vi "Curtin1.vi"() -> ()   [LabVIEW 2022 SP3]
uses:
  ViolinSubs/Curtin1_Label.ctl
  ViolinSubs/GraphType.ctl
  <vilib>/Utility/miscctls.llb/LVPoint32TypeDef.ctl
  ViolinSubs/Mic/Mic_Global.vi
  ViolinSubs/Perspective/subs/Perspective_Globals.vi
  <vilib>/Platform/browser.llb/Open URL in Default Browser (string).vi
panel:
  in  "microphone":bool
  in  "Device":u16(ring) items=["BuerginBase Microphone", "MacBook Pro Microphone", "Microsoft Teams Audio"]
  out "comma?":bool
  out "startX":i32
  out "Ctrl":bool
  out "beta":string
  in  "Settings":u16(ring) items=["Settings...", "Preferences", "Templates", "Calibrations", "Live View", "Motor Cntrl"]
  in  "ScratchPads":u16(ring) items=["Scratch...", "Admittance Scratchpad", "Radiation ScratchPad", "ScratchPad", "TapTones ScratchPad"]
  in  "New Test":u16(ring) items=["New Test...", "Admittance H", "JC H 12 radiation", "JC H 7 radiation", "JC HV 24 radiation", "TEST"]
  in  "Help":bool
  in  "About":bool
  in  "Start":bool
  in  "email":bool
  in  "Interpret":bool
  in  "Force YRescale":bool
  out "Complex Out":cluster{dbl, "df":dbl, cdb[]}[](array[cluster])
  out "# selected":i32
  in  "Fun":bool
  out "Version":string
  in  "Preferences":bool
  in  "Set Colors":bool
  in  "Colors":u16(ring) items=["Name Current...", "Last Saved", "24 Colors", "rear"]
  in  "Share":bool
  in  "Undo":bool
  in  "Clear All":bool
  in  "select all":bool
  in  "deselect":bool
  in  "Clear":bool
  in  "Lists":bool
  in  "Browse":bool
  in  "Search":bool
  in  "Redo":bool
  in  "Files":T1[](array[typedef])
  in  "zoom":bool
  in  "Mouse Down?":bool
  in  "Views":T3={"View Type"=0, "Smoothing"=0, "Bands"=0, "Edit"=FALSE, "rescale Y"=FALSE, "rescale X"=FALSE, "X_Low"=0.0, "X_High"=0.0, "dB Range"=40.0, "Excel"=FALSE, "Y Scaling"=TRUE, "X Scaling"=TRUE, "Plot"=0} {"Plot" items=["FRF", "rad phase unwrapped", "deg phase unwrapped", "rad phase wrapped", "deg phase wrapped", "White Plots", "MJ Map", "Real and Imaginary"]; "Bands" items=["No Bands", "JC violin 200-7000 Flat (200-7000)", "JC violin (200-780-1740-2930-7000)", "JC violin (200-780-7000)"]; "Smoothing" items=["No smoothing"=0, "1/4 semitone"=25, "1/2 semitone"=50, "1 semitone"=100, "2 semitones"=200, "3 semitones"=300, "4 semitones"=400, "Octave"=1200, "Woodhouse"=19]; "View Type" items=["As measured"=0, "Normalize"=1, "Cplx Average"=3, "Real Average"=4, "Standard Deviation"=5]}
  out "Position":string
  in  "Color Table":T4(ring)=enum."Greyscale"
  out "MJPlot":dbl[][](graph)
  out "Coords":T5
  out "White Plots":picture
  out "FRF":cluster{"x0":dbl, "df":dbl, dbl[]}[](graph)
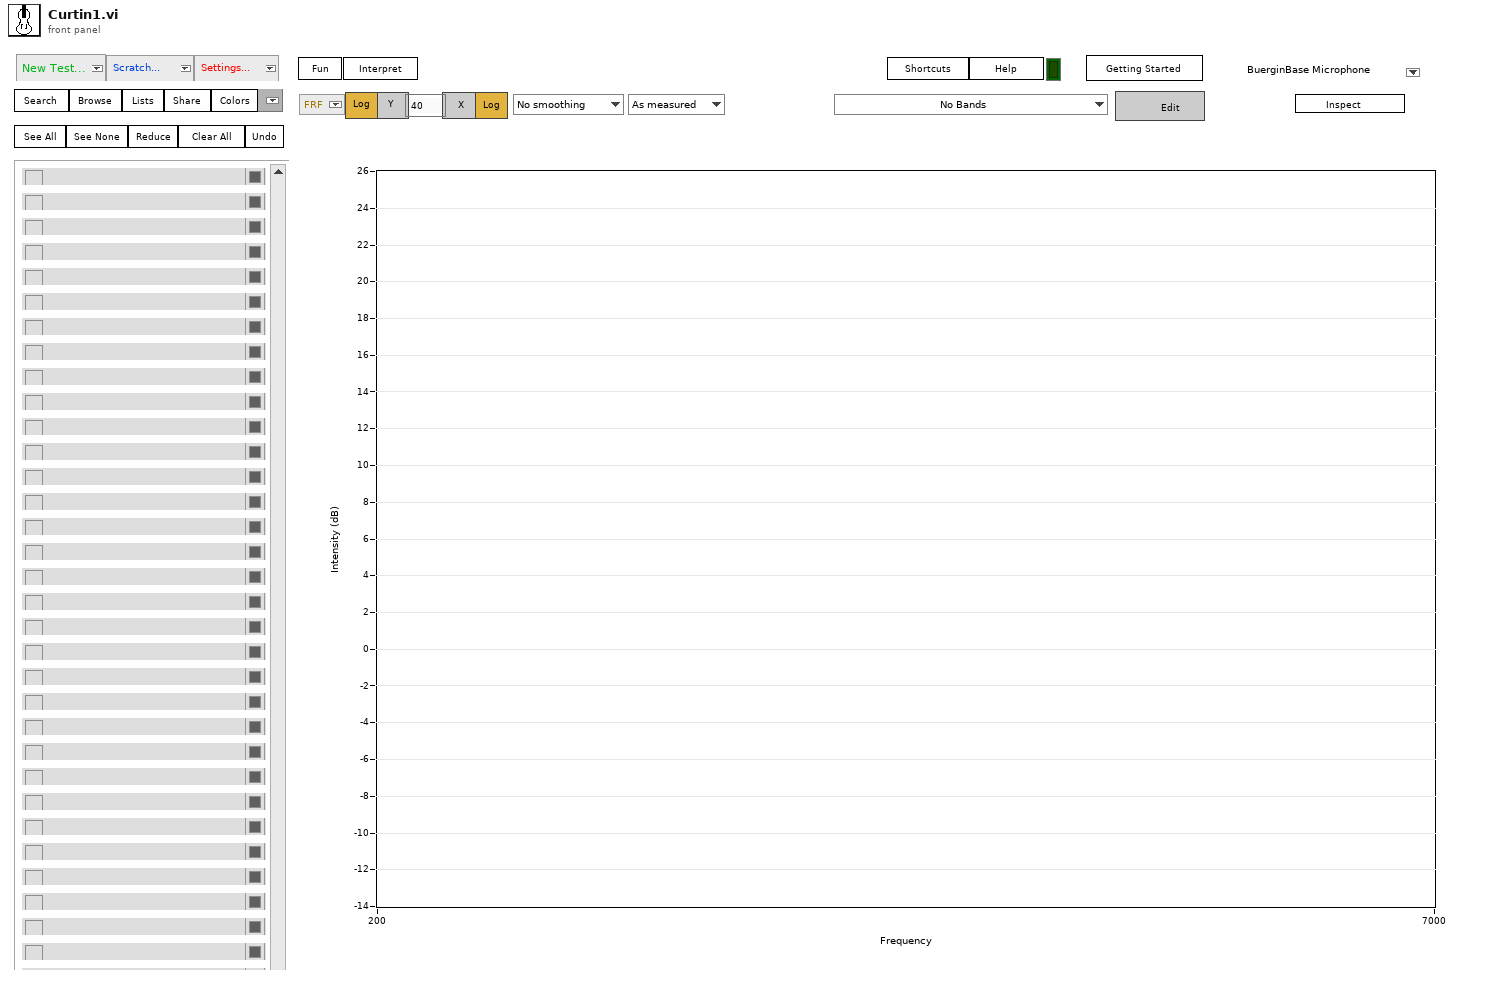
[diagram p1: front panel]
types:
  T1 = typedef "Curtin1_Label.ctl" = cluster{"Show?":bool, "Name":string, "Color":u32, "Path":path, "Show Notes":bool}
  T2 = typedef "GraphType.ctl" = u16
  T3 = cluster{"View Type":u16, "Smoothing":u16, "Bands":u16, "Edit":bool, "rescale Y":bool, "rescale X":bool, "X_Low":dbl, "X_High":dbl, "dB Range":dbl, "Excel":bool, "Y Scaling":bool, "X Scaling":bool, "Plot":T2}
  T4 = enum16{"Apricot", "Carnation", "Ether", "Greyscale", "Greyscale-banded", "Hot Metal", "Lava Waves", "Mac", "Morning Glory", "Rainbow", "Rainbow-banded", "Rainbow-inverted", "Rainbow-striped", "Saturn", "Seismic", "Space"}
  T5 = typedef "LVPoint32TypeDef.ctl" = cluster{"Horizontal":i32, "Vertical":i32}
  T6 = enum32{"SPL", "Voltage", "Accelerometer", "Vibrometer", "home", "Units"}
  T7 = enum16{"big-endian, network order", "native, host order", "little-endian"}
  T8 = enum16{"Grab Lines", "Grab Bands", "Grab Centroids"}
  T9 = cluster{"Alerts":bool, "Log X Axis":bool, "dB scale":bool, "Averaging":bool, "Fade":dbl, "Centroids?":bool}
  T10 = typedef "LVBoundsTypeDef.ctl" = cluster{"Width":u32, "Height":u32}
  T11 = typedef "LVPositionTypeDef.ctl" = cluster{"Left":i32, "Top":i32}
  T12 = typedef "PreferencesControl.ctl" = cluster{"Name of test":string, "Date":timestamp, "Location":string, "Template":string, "Soundcard":string, "resolution":u16, "Sampling rate":u16, "Ch1 Gain ":dbl, "Ch2 Gain":dbl, "Sample time (s)":dbl, "Pre-trigger (s)":dbl, "Hammer Threshold":dbl, "Positions":i16, "Taps/Position":i16, "Set Names":string, "Freq resolution":dbl, "Hammer cutoff":dbl, "Mic cutoff":dbl, "Double bounce ":dbl, "Hammer Cal":dbl, "dB Offset":dbl, "Accel Cal":dbl, "Vibrometer Cal":dbl, "Mic Cal":dbl, "Output":u16, "Voltage Cal":dbl, "Vibrometer Port":refnum<visa-resource-name>, "Range":u16, "High Pass":u16, "Bandwidth":u16, "X Range":cluster{"Minimum":dbl, "Maximum":dbl, "Increment":dbl, "Minor Increment":dbl, "Start":dbl}[], "Y Range":cluster{"Minimum":dbl, "Maximum":dbl, "Increment":dbl, "Minor Increment":dbl, "Start":dbl}[], "dB Spread":dbl, "Trigger":u16, "Ch_1":u8, "Ch_2":u8, "flip?":bool, "60Hz":bool, "Time offset":dbl, "Piezo Cal":dbl, "Default Notes":string}
  T13 = typedef "eventvkey.ctl" = enum16{"ASCII", "Enter", "Return", "Shift", "Ctrl", "Alt", "Cmd", "Opt", "Caps", "NumLock", "Clear", "Break", "Up", "Down", "Left", "Right", "Insert", "Delete", "Home", "End", "PageUp", "PageDown", "Escape", "Help", "Pause", "ScrollLock", "F1", "F2", "F3", "F4", "F5", "F6", "F7", "F8", "F9", "F10", "F11", "F12", "F13", "F14", "F15", "F16", "F17", "F18", "F19", "F20", "F21", "F22", "F23", "F24", "Play", "VolumeUp", "VolumeDown", "Mute", "Two Byte Char"}
  T14 = typedef "LVMouseTypeDef.ctl" = cluster{"Mouse Position":cluster{"X":i32, "Y":i32}, "Mouse Modifiers":cluster{"Button Down":bool, "Shift Mod":bool, "Menu Mod":bool, "Option Mod":bool}}
  T15 = enum32{"Invalid", "Standard", "Closed", "Hidden", "Minimized", "Maximized"}
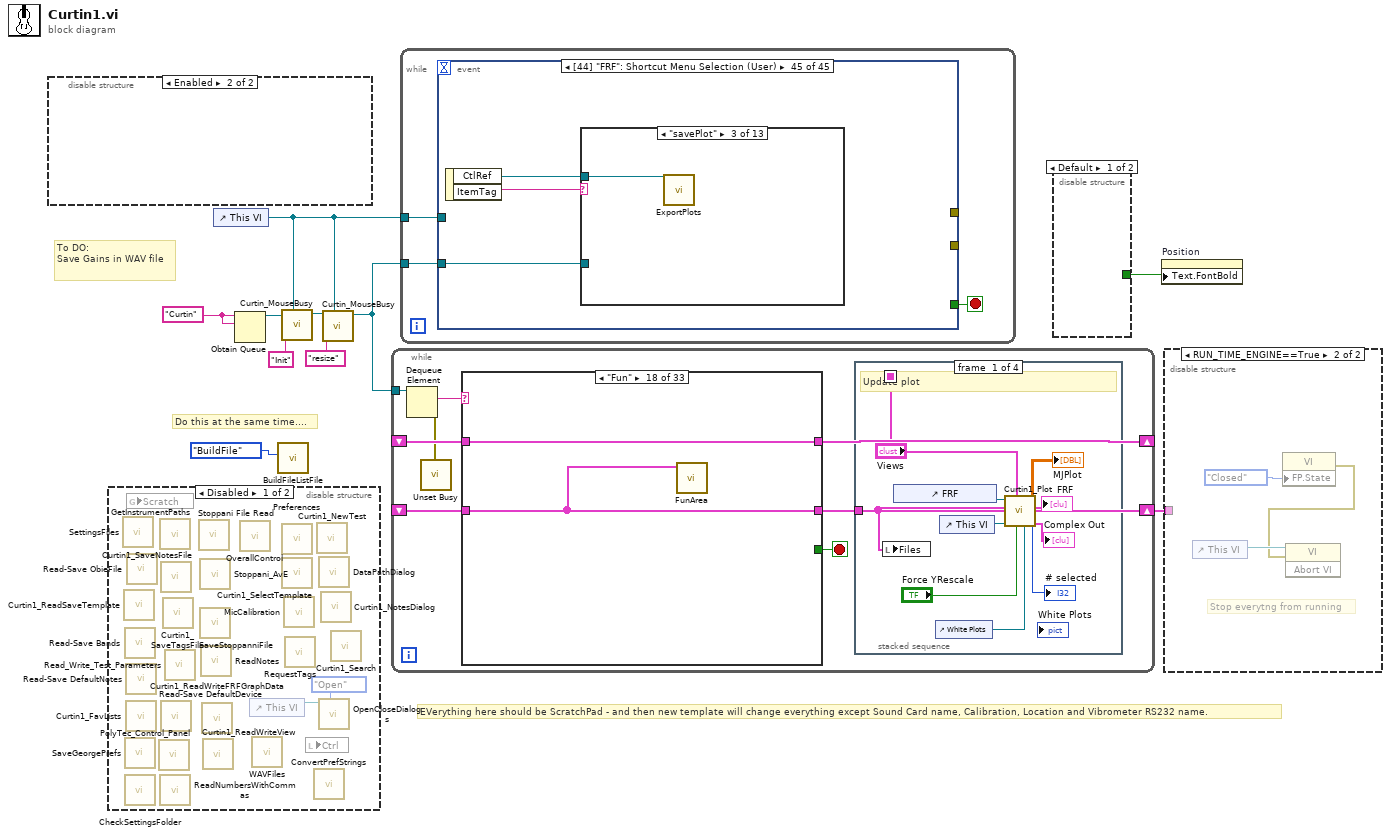
[diagram p0: block diagram]
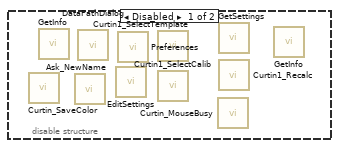
[diagram p2: hidden frame]
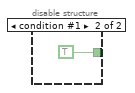
[diagram p4: hidden frame]
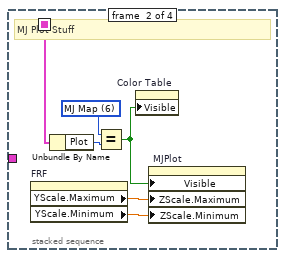
[diagram p6: hidden frame]
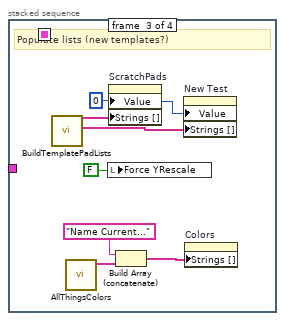
[diagram p7: hidden frame]
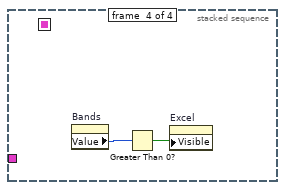
[diagram p8: hidden frame]
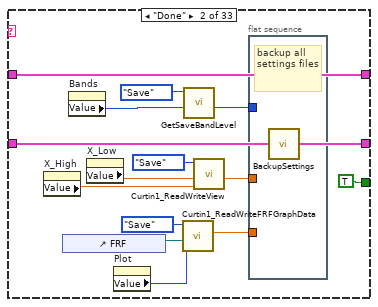
[diagram p10: hidden frame]
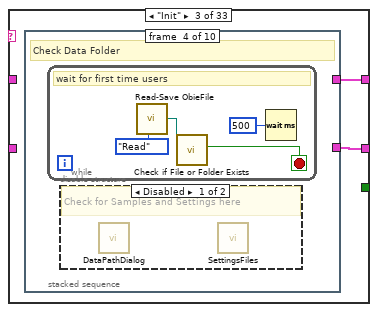
[diagram p11: hidden frame]
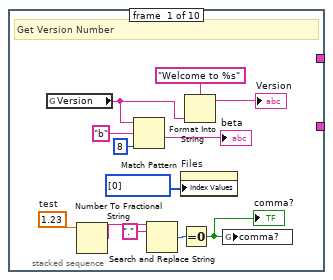
[diagram p12: hidden frame]
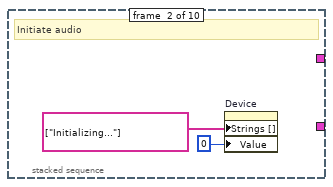
[diagram p13: hidden frame]
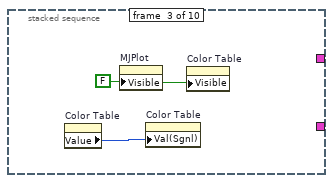
[diagram p14: hidden frame]
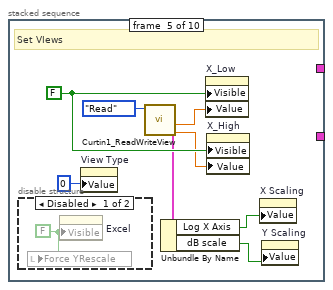
[diagram p16: hidden frame]
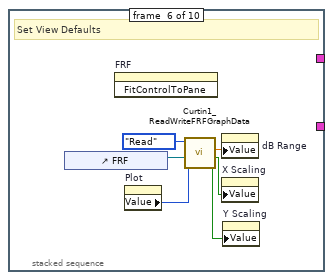
[diagram p18: hidden frame]
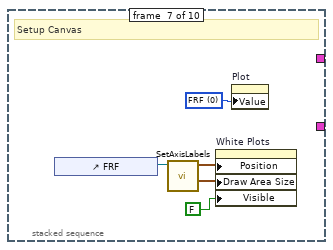
[diagram p19: hidden frame]
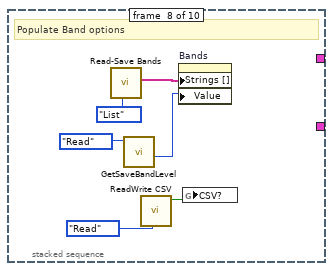
[diagram p20: hidden frame]
diagram:
  w8 = "Curtin" ("name (unnamed)")
  # "Do this at the same time...."
  # "To DO:\nSave Gains in WAV file"
  # "EVerything here should be ScratchPad - and then new template will change everything except Sound Card name, Calibration, Location and Vibrometer RS232 name."
  n1 = disable-structure shown="Enabled" {
    frame Disabled {
      n2 = call "Curtin_SaveColor.vi"() -> ()  [unwired: 10 in, 2 out]
      n3 = call "GetInfo.vi"() -> ()  [unwired: 11 in, 1 out]
      n4 = call "Ask_NewName.vi"() -> ()  [unwired: 10 in, 2 out]
      n5 = call "DataPathDialog.vi"() -> ()  [unwired: 10 in, 2 out]
      n6 = call "EditSettings.vi"() -> ()  [unwired: 10 in, 2 out]
      n7 = call "Preferences.vi"() -> ()  [unwired: 9 in, 3 out]
      n8 = call "Curtin1_SelectTemplate.vi"() -> ()  [unwired: 10 in, 2 out]
      n9 = call "Curtin1_SelectCalib.vi"() -> ()  [unwired: 11 in, 1 out]
      n10 = call "Curtin_MouseBusy.vi"() -> ()  [unwired: 11 in, 1 out]
      n11 = call "GetSettings.vi"() -> ()  [unwired: 10 in, 2 out]
      n12 = call "Curtin1_Recalc.vi"() -> ()  [unwired: 12 in]
      n13 = call "GetInfo.vi"() -> ()  [unwired: 11 in, 1 out]
    }
    frame Enabled {
    }
  }
  n14 = disable-structure shown="Disabled" {
    frame Disabled {
      n15 = call "SettingsFiles.vi"() -> ()  [unwired: 10 in, 2 out]
      n16 = call "Curtin1_ReadSaveTemplate.vi"() -> ()  [unwired: 8 in, 4 out]
      n17 = call "Read-Save Bands.vi"() -> ()  [unwired: 8 in, 4 out]
      n18 = call "SaveGeorgePrefs.vi"() -> ()  [unwired: 10 in, 2 out]
      n19 = call "CheckSettingsFolder.vi"() -> ()  [unwired: 12 in]
      n20 = call "Read-Save DefaultNotes.vi"() -> ()  [unwired: 10 in, 2 out]
      n21 = call "Curtin1_FavLists.vi"() -> ()  [unwired: 8 in, 4 out]
      n22 = global read "Mic_Global.vi" "Scratch"() -> ()  [unwired: 1 in]
      n23 = call "Read-Save ObieFile.vi"() -> ()  [unwired: 9 in, 3 out]
      n24 = call "PolyTec_Control_Panel.vi"() -> ()  [unwired: 9 in, 3 out]
      n25 = call "GetInstrumentPaths.vi"() -> ()  [unwired: 7 in, 5 out]
      n26 = call "ReadNumbersWithCommas.vi"() -> ()  [unwired: 8 in, 4 out]
      n27 = call "Curtin1_SaveNotesFile.vi"() -> ()  [unwired: 12 in]
      n28 = call "Read-Save DefaultDevice.vi"() -> ()  [unwired: 10 in, 2 out]
      n29 = call "Curtin1_SaveTagsFile.vi"() -> ()  [unwired: 12 in]
      n30 = call "Read_Write_Test_Parameters.vi"() -> ()  [unwired: 10 in, 2 out]
      n31 = call "Stoppani File Read.vi"() -> ()  [unwired: 3 in, 4 out]
      n32 = call "Stoppani_AvE.vi"() -> ()  [unwired: 8 in, 4 out]
      n33 = call "SaveStoppanniFile.vi"() -> ()  [unwired: 11 in, 1 out]
      n34 = call "ReadNotes.vi"() -> ()  [unwired: 10 in, 2 out]
      n35 = call "Curtin1_ReadWriteFRFGraphData.vi"() -> ()  [unwired: 9 in, 3 out]
      n36 = call "Curtin1_ReadWriteView.vi"() -> ()  [unwired: 9 in, 3 out]
      n37 = call "OverallControl.vi"() -> ()  [unwired: 10 in, 2 out]
      n38 = control-ref of="This VI"() -> (w11:refnum<vi>)
      n39 = call "WAVFiles.vi"() -> ()  [unwired: 8 in, 4 out]
      n40 = call "Preferences.vi"() -> ()  [unwired: 9 in, 3 out]
      n41 = call "Curtin1_SelectTemplate.vi"() -> ()  [unwired: 10 in, 2 out]
      n42 = call "MicCalibration.vi"() -> ()  [unwired: 11 in, 1 out]
      n43 = call "RequestTags.vi"() -> ()  [unwired: 11 in, 1 out]
      n44 = local read "Ctrl"() -> ()  [unwired: 1 in]
      n45 = call "ConvertPrefStrings.vi"() -> ()  [unwired: 10 in, 2 out]
      n46 = call "Curtin1_NewTest.vi"() -> ()  [unwired: 10 in, 2 out]
      n47 = call "DataPathDialog.vi"() -> ()  [unwired: 10 in, 2 out]
      n48 = call "OpenCloseDialogs.vi"("Task"=enum16{"Open", "Close"}."Open", "VI in"=w11) -> ()  [unwired: 8 in, 2 out]
      n49 = call "Curtin1_NotesDialog.vi"() -> ()  [unwired: 9 in, 3 out]
      n50 = call "Curtin1_Search.vi"() -> ()  [unwired: 10 in, 2 out]
    }
    frame Enabled {
    }
  }
  n51 = control-ref of="This VI"() -> (w2:refnum<vi>)
  n52 = Obtain Queue(name (unnamed)=w8, element data type=w8) -> (queue out=w7:refnum<queue>)  [unwired: 3 in, 2 out]
  n53 = call "BuildFileListFile.vi"("Task"=enum16{"BuildFile", "ReadFile"}."BuildFile") -> ()  [unwired: 9 in, 2 out]
  n54 = call "Curtin_MouseBusy.vi"("VI in"=w2, "element"="Init", "queue in"=w7) -> ("queue out"=w4:refnum<queue>)  [unwired: 8 in]
  n55 = call "Curtin_MouseBusy.vi"("VI in"=w2, "element"="resize", "queue in"=w4) -> ("queue out"=w5:refnum<queue>)  [unwired: 8 in]
  n56 = while {
    tunnel: w5 -> [w19]
    shift-right: [w16] -> w9
    shift-left: _ -> [w17]
    shift-right: [w14] -> _
    shift-left: _ -> [w15]
    stop <- w18 stop-if-true
    n57 = Dequeue Element(queue=w19) -> (element=w20:string, error out=w13:errorcluster)  [unwired: 2 in, 2 out]
    n58 = call <vilib>:"Unset Busy.vi"("error in (no error)"=w13) -> ()  [unwired: 10 in, 1 out]
    n59 = case shown="\"Fun\"" w20 {
      selector: w20 -> [_ _ _ _ _ _ _ _ _ _ _ _ _ _ _ _ _ _ _ _ _ _ _ _ _ _ _ _ _ _ w300 _ _]
      tunnel: [_ TRUE ("Discard?") _ _ _ _ _ _ _ _ _ _ _ _ _ _ _ _ _ _ _ _ _ _ _ _ _ _ _ _ _ _ _] -> w18
      tunnel: w17 -> [w47 w60 _ _ w128 w137 w153 w158 w160 w162 w164 w177 w184 w189 w200 w209 w221 w225 w227 w229 w233 w238 w241 w244 w257 w269 w275 w280 w285 w290 w301 w308 w331]
      tunnel: [w47 w60 w62 w116 w128 w139 w153 w158 w160 w162 w168 w176 w185 w191 w195 w209 w220 w225 w227 w229 w231 w237 w240 w244 w256 w268 w274 w282 T1[] [] ("Files") w292 w301 w308 w331] -> w16
      tunnel: [w46 w59 w63 w117 w131 w141 w154 w159 w161 w163 w166 w178 w186 w192 w201 w210 w223 w226 w228 w230 w234 w239 w242 w245 w258 w267 w273 w279 w286 w293 w302 w312 w332] -> w14
      tunnel: w15 -> [w46 w59 _ w118 w131 w141 w154 w159 w161 w163 w167 w179 w187 w193 w202 w210 w224 w226 w228 w230 w235 w239 w242 w245 w259 w267 w273 w281 w288 w291 w302 w312 w332]
      frame Default {
      }
      frame "Done" {
        n60 = property on="X_High" class="DigNum (strict)"() -> ("Value"=w54:dbl)  [unwired: 2 in, 2 out]
        n61 = control-ref of="FRF"() -> (w57:refnum<vi>)
        n62 = property on="Bands" class="Ring (strict)"() -> ("Value"=w52:u16)  [unwired: 2 in, 2 out]
        n63 = property on="X_Low" class="DigNum (strict)"() -> ("Value"=w55:dbl)  [unwired: 2 in, 2 out]
        n64 = property on="Plot" class="Ring (strict)"() -> ("Value"=w48:T2)  [unwired: 2 in, 2 out]
        n65 = call "Curtin1_ReadWriteFRFGraphData.vi"("Type"=w48, "FRF"=w57, "Task"=enum16{"Read", "Save"}."Save") -> ("dB"=w49:dbl)  [unwired: 6 in, 2 out]
        n66 = call "GetSaveBandLevel.vi"("Value in"=w52, "Task"=enum16{"Read", "Save"}."Save") -> ("Value out"=w51:u16)  [unwired: 9 in]
        n67 = call "Curtin1_ReadWriteView.vi"("X_High"=w54, "X_Low"=w55, "Task"=enum16{"Read", "Save"}."Save") -> ("X_Low out"=w50:dbl)  [unwired: 6 in, 2 out]
        n68 = flat-sequence {
          tunnel: w51 -> [_]
          tunnel: w50 -> [_]
          tunnel: w49 -> [_]
          frame #0 {
            # "backup all settings files"
            n69 = call "BackupSettings.vi"() -> ()  [unwired: 12 in]
          }
        }
      }
      frame "Init" {
        n70 = stacked-sequence {
          tunnel: [_ _ _ _ _ _ _ _ _ cluster{"files":T1[]}[] [] ("Array in")] -> w63
          tunnel: [_ _ _ _ _ _ _ _ _ T1[] [] ("Files")] -> w62
          frame #0 {
            w65 = 1.23  # test
            # "Get Version Number"
            n71 = global read "Mic_Global.vi" "Version"() -> (w69:string)
            n72 = Number To Fractional String(number=w65) -> (F-format string=w64:string)  [unwired: 3 in]
            n73 = Match Pattern(string=w69, regular expression="b", offset (0)=8) -> (after substring=→"beta":string)  [unwired: 3 out]
            n74 = Search and Replace String(input string=w64, search string=".") -> (number of replacements=w68:i32)  [unwired: 6 in, 3 out]
            n75 = property on="Files" class="Arr"("Index Values"=u32[] [0]) -> ()  [unwired: 2 in, 2 out]
            n76 = Equal To 0?(x=w68) -> (x = 0?=w66:bool)
            "comma?" <- w66
            n77 = Format Into String(format string="Welcome to %s", w69) -> (resulting string=→"Version":string)  [unwired: 2 in, 1 out]
            n78 = global write "Mic_Global.vi" "comma?"(w66) -> ()
          }
          frame #1 {
            # "Initiate audio"
            n79 = property on="Device" class="Ring (strict)"("Strings []"=string[] ["Initializing..."] ("Strings [4]"), "Value"=0) -> ()  [unwired: 2 in, 2 out]
          }
          frame #2 {
            w79 = FALSE ("Visible")
            n80 = property on="Color Table" class="Enum (strict)"() -> ("Value"=w78:T4)  [unwired: 2 in, 2 out]
            n81 = property on="MJPlot" class="IntGraph (strict)"("Visible"=w79) -> ()  [unwired: 2 in, 2 out]
            n82 = property on="Color Table" class="Enum (strict)"("Val(Sgnl)"=w78) -> ()  [unwired: 2 in, 2 out]
            n83 = property on="Color Table" class="Enum (strict)"("Visible"=w79) -> ()  [unwired: 2 in, 2 out]
          }
          frame #3 {
            # "Check Data Folder"
            n84 = while {
              stop <- w81 stop-if-true
              # "wait for first time users"
              n85 = call "Read-Save ObieFile.vi"("Task"=enum16{"Save", "Read"}."Read") -> ("DataPath Out"=w83:path)  [unwired: 8 in, 2 out]
              n86 = call <vilib>:"Check if File or Folder Exists.vi"("path"=w83) -> ("file or folder exists?"=w81:bool)  [unwired: 8 in, 2 out]
              n87 = Wait (ms)(milliseconds to wait=u32 500) -> ()  [unwired: 1 out]
            }
            n88 = disable-structure shown="Disabled" {
              frame Disabled {
                # "Check for Samples and Settings here"
                n89 = call "DataPathDialog.vi"() -> ()  [unwired: 10 in, 2 out]
                n90 = call "SettingsFiles.vi"() -> ()  [unwired: 10 in, 2 out]
              }
              frame Enabled {
              }
            }
          }
          frame #4 {
            w91 = FALSE ("Visible")
            # "Set VIews"
            n91 = disable-structure shown="Disabled" {
              frame Disabled {
                w92 = FALSE ("Visible")
                n92 = local write "Force YRescale"(w92) -> ()
                n93 = property on="Excel" class="Bool"("Visible"=w92) -> ()  [unwired: 2 in, 2 out]
              }
              frame Enabled {
              }
            }
            n94 = property on="View Type" class="Ring (strict)"("Value"=u16 0) -> ()  [unwired: 2 in, 2 out]
            n95 = call "Curtin1_ReadWriteView.vi"("Task"=enum16{"Read", "Save"}."Read") -> ("X_High out"=w88:dbl, "X_Low out"=w89:dbl, "View"=w84:T9)  [unwired: 8 in]
            n96 = Unbundle By Name(w84) -> ("Log X Axis"=w85:bool, "dB scale"=w86:bool)
            n97 = property on="X_Low" class="DigNum (strict)"("Visible"=w91, "Value"=w89) -> ()  [unwired: 2 in, 2 out]
            n98 = property on="X_High" class="DigNum (strict)"("Visible"=w91, "Value"=w88) -> ()  [unwired: 2 in, 2 out]
            n99 = property on="X Scaling" class="Bool (strict)"("Value"=w85) -> ()  [unwired: 2 in, 2 out]
            n100 = property on="Y Scaling" class="Bool (strict)"("Value"=w86) -> ()  [unwired: 2 in, 2 out]
          }
          frame #5 {
            # "Set View Defaults"
            n101 = control-ref of="FRF"() -> (w98:refnum<vi>)
            n102 = invoke on="FRF" class="WFGraph (strict)" method="FitControlToPane"() -> ()  [unwired: 3 in, 3 out]
            n103 = property on="Plot" class="Ring (strict)"() -> ("Value"=w95:T2)  [unwired: 2 in, 2 out]
            n104 = call "Curtin1_ReadWriteFRFGraphData.vi"("Type"=w95, "FRF"=w98, "Task"=enum16{"Read", "Save"}."Read") -> ("y log?"=w94:bool, "x log?"=w93:bool, "dB"=w96:dbl)  [unwired: 6 in]
            n105 = property on="dB Range" class="DigNum (strict)"("Value"=w96) -> ()  [unwired: 2 in, 2 out]
            n106 = property on="X Scaling" class="Bool (strict)"("Value"=w93) -> ()  [unwired: 2 in, 2 out]
            n107 = property on="Y Scaling" class="Bool (strict)"("Value"=w94) -> ()  [unwired: 2 in, 2 out]
          }
          frame #6 {
            w99 = T2 0 items=["FRF", "rad phase unwrapped", "deg phase unwrapped", "rad phase wrapped", "deg phase wrapped", "White Plots"] ("Value")
            # "Setup Canvas"
            n108 = control-ref of="FRF"() -> (w103:refnum<vi>)
            n109 = call "SetAxisLabels.vi"("WaveformGraph in"=w103) -> ("Bounds"=w101:T10, "Position"=w102:T11)  [unwired: 8 in, 1 out]
            n110 = property on="White Plots" class="Pict"("Position"=w102, "Draw Area Size"=w101, "Visible"=FALSE) -> ()  [unwired: 2 in, 2 out]
            n111 = property on="Plot" class="Ring (strict)"("Value"=w99) -> ()  [unwired: 2 in, 2 out]
          }
          frame #7 {
            # "Populate Band options"
            n112 = call "Read-Save Bands.vi"("Task"=enum16{"Save", "Read", "List"}."List") -> ("Long names"=w109:string[])  [unwired: 7 in, 3 out]
            n113 = call "GetSaveBandLevel.vi"("Task"=enum16{"Read", "Save"}."Read") -> ("Value out"=w106:u16)  [unwired: 10 in]
            n114 = call "ReadWrite CSV.vi"("Task"=enum16{"Save", "Read"}."Read") -> ("csv Out"=w104:bool)  [unwired: 10 in]
            n115 = property on="Bands" class="Ring (strict)"("Strings []"=w109, "Value"=w106) -> ()  [unwired: 2 in, 2 out]
            n116 = global write "Mic_Global.vi" "CSV?"(w104) -> ()
          }
          frame #8 {
            # "Always start everyone with ScratchPad \n\nRead the latest calibration but do not \ndo anything with it (no error code/saving)"
            # "Upload  ScratchPad template"
            n117 = call "UpdateScratchPad.vi"() -> ("Settings Out"=w111:T12)  [unwired: 10 in, 1 out]
            n118 = global write "Mic_Global.vi" "Settings"(w111) -> ()
            n119 = control-ref of="Device"() -> (w112:refnum<vi>)
            n120 = call "Curtin1_soundcards.vi"("hush?"=TRUE, "Settings In"=w111, "device:"=w112) -> ()  [unwired: 7 in, 2 out]
          }
          frame #9 {
            # "Initialize Undo and List"
          }
        }
      }
      frame "Update" {
        # "NOTE: info box is in this frame"
        n121 = call "Curtin1_NotesDialog.vi"("Files"="Files") -> ("Color"=w120:u32[], "removed?"=w119:bool, "Array"=w116:T1[])  [unwired: 8 in]
        n122 = call "Curtin1_Color.vi"("Color"=w120) -> ()  [unwired: 9 in, 2 out]
        n123 = case shown="True" w119 {
          tunnel: w118 -> [w122 w125]
          tunnel: [w122 w124] -> w117
          tunnel: w116 -> [_ w123]
          frame False {
          }
          frame True {
            # "removed a plot"
            n124 = call "Curtin_Undo.vi"("New Files"=w123, "Array in"=w125) -> ("Array out"=w124:cluster{"files":T1[]}[])  [unwired: 9 in]
          }
        }
        n125 = property on="Colors" class="Ring (strict)"("Value"=-1) -> ()  [unwired: 2 in, 2 out]
      }
      frame "Zoom" {
        n126 = for {
          tunnel: w128 -> [w134] mode=indexing
          tunnel: [w133] -> w127 mode=indexing if=w132
          n127 = Unbundle By Name(w134) -> ("Name"=w133:string, "Show?"=w132:bool)
        }
        n128 = property on="Plot" class="Ring (strict)"() -> ("Value"=w126:T2)  [unwired: 2 in, 2 out]
        n129 = property on="dB Range" class="DigNum (strict)"() -> ("Value"=w129:dbl)  [unwired: 2 in, 2 out]
        n130 = control-ref of="FRF"() -> (w130:refnum<vi>)
        n131 = call "GraphZoom.vi"("Plot"=w126, "Names"=w127, "dB Range"=w129, "Graph"=w130) -> ()  [unwired: 8 in]
      }
      frame "Preferences" {
        n132 = control-ref of="Files"() -> (w140:refnum<vi>)
        n133 = call "Preferences.vi"("FileList"=w140, "Files"=w137) -> ("Settings out"=w135:T12, "Success?"=w138:bool, "Fixed Files"=w136:T1[])  [unwired: 7 in]
        n134 = case shown="True" w138 {
          tunnel: w136 -> [_ w150]
          tunnel: [w142 w150] -> w139
          tunnel: w137 -> [w142 _]
          tunnel: w135 -> [_ w146]
          frame False {
          }
          frame True {
            n135 = global read "Mic_Global.vi" "View"() -> (w149:T9)
            n136 = call "UpdateScratchPad.vi"("Settings"=w146) -> ("Settings Out"=w143:T12)  [unwired: 9 in, 1 out]
            n137 = Unbundle By Name(w149) -> ("Log X Axis"=w148:bool, "dB scale"=w147:bool)
            n138 = control-ref of="Device"() -> (w145:refnum<vi>)
            n139 = call "Curtin1_soundcards.vi"("hush?"=TRUE, "Settings In"=w143, "device:"=w145) -> ()  [unwired: 7 in, 2 out]
            n140 = property on="X Scaling" class="Bool (strict)"("Value"=w148) -> ()  [unwired: 2 in, 2 out]
            n141 = property on="Y Scaling" class="Bool (strict)"("Value"=w147) -> ()  [unwired: 2 in, 2 out]
          }
        }
      }
      frame "Templates" {
        n142 = global read "Mic_Global.vi" "Scratch"() -> (w152:string)
        n143 = call "EditSettings.vi"("Template in"=w152) -> ("Settings out"=w151:T12)  [unwired: 9 in, 1 out]
        n144 = call "UpdateScratchPad.vi"("Settings"=w151) -> ()  [unwired: 9 in, 2 out]
      }
      frame "Calibrations" {
        # "Saves a new calib file\nand it is pushed in test"
        n145 = call "UpdateScratchPad.vi"() -> ("Settings Out"=w156:T12)  [unwired: 10 in, 1 out]
        n146 = call "MicCalibration.vi"("Type"=T6."home" ("Tyoe"), "Settings"=w156) -> ("Settings Out"=w155:T12)  [unwired: 9 in]
        n147 = global write "Mic_Global.vi" "Settings"(w155) -> ()
        n148 = call "UpdateScratchPad.vi"("Settings"=w155) -> ()  [unwired: 9 in, 2 out]
      }
      frame "LiveView" {
        n149 = call "LiveSignal.vi"() -> ()  [unwired: 12 in]
      }
      frame "MotorControl" {
        n150 = call "MotorControl.vi"() -> ()  [unwired: 12 in]
      }
      frame "Browse" {
        n151 = Array Size(array=w164) -> (size(s)=w165:i32)
        n152 = case shown="0" w165 {
          frame Default {
          }
          frame 0 {
            n153 = local write "Force YRescale"(TRUE ("Force YRescale")) -> ()
          }
        }
        n154 = call "Curtin_Undo.vi"("New Files"=w164, "Array in"=w167) -> ("Array out"=w166:cluster{"files":T1[]}[])  [unwired: 9 in]
        n155 = call "Curtin1_LoadFile.vi"("Files in"=w164) -> ("Files out"=w168:T1[])  [unwired: 10 in]
      }
      frame "Preload" {
        n156 = call "Curtin1_GlobalFolder.vi"() -> ("Samples"=w170:path)  [unwired: 1 in, 1 out]
        n157 = List Folder(path=w170, pattern="*.AvC") -> (path out=w173:path, filenames=w172:string[])  [unwired: 2 in, 2 out]
        n158 = call "Curtin_Undo.vi"("New Files"=w177, "Array in"=w179) -> ("Array out"=w178:cluster{"files":T1[]}[])  [unwired: 9 in]
        n159 = local write "Force YRescale"(TRUE ("Force YRescale")) -> ()
        n160 = for {
          tunnel: w173 -> [w182]
          tunnel: w172 -> [w181] mode=indexing
          tunnel: [w180] -> w171 mode=indexing
          n161 = Build Path(base path=w182, name or relative path=w181) -> (appended path=w180:path)
        }
        n162 = call "Curtin1_AddTest.vi"("Selected Paths"=w171) -> ("New Files"=w176:T1[])  [unwired: 10 in]
      }
      frame "Search" {
        n163 = Array Size(array=w184) -> (size(s)=w183:i32)
        n164 = case shown="0" w183 {
          frame Default {
          }
          frame 0 {
            n165 = local write "Force YRescale"(TRUE ("Force YRescale")) -> ()
          }
        }
        n166 = call "Curtin_Undo.vi"("New Files"=w184, "Array in"=w187) -> ("Array out"=w186:cluster{"files":T1[]}[])  [unwired: 9 in]
        n167 = call "Curtin1_Search.vi"("Old Files"=w184) -> ("New Files"=w185:T1[])  [unwired: 9 in, 1 out]
      }
      frame "Lists" {
        n168 = Array Size(array=w189) -> (size(s)=w190:i32)
        n169 = case shown="0" w190 {
          frame Default {
          }
          frame 0 {
            n170 = local write "Force YRescale"(TRUE ("Force YRescale")) -> ()
          }
        }
        n171 = call "Curtin_Undo.vi"("New Files"=w189, "Array in"=w193) -> ("Array out"=w192:cluster{"files":T1[]}[])  [unwired: 9 in]
        n172 = call "Curtin1_Lists.vi"("Old Files"=w189) -> ("New Files"=w191:T1[])  [unwired: 10 in]
      }
      frame "newColors" {
        n173 = property on="Colors" class="Ring (strict)"() -> ("Strings []"=w198:string[], "Value"=w199:u16)  [unwired: 2 in, 2 out]
        n174 = Index Array(array=w198, index=w199) -> (element=w197:string)
        n175 = call "AllThingsColors.vi"("Choice"=w197) -> ("Possible Colors"=w196:string[])  [unwired: 10 in]
        n176 = for {
          tunnel: w200 -> [w206] mode=indexing
          tunnel: [w205] -> w195 mode=indexing
          tunnel: w196 -> [_]
          i -> [w204]
          n177 = call "Curtin1_Color.vi"("Offset"=w204) -> ("New color"=w203:u32)  [unwired: 9 in, 1 out]
          n178 = Bundle By Name(cluster=w206, "Color"=w203) -> (w205:T1)
        }
        n179 = call "Curtin_Undo.vi"("New Files"=w200, "Array in"=w202) -> ("Array out"=w201:cluster{"files":T1[]}[])  [unwired: 9 in]
        n180 = local write "Files"(w195) -> ()
      }
      frame "saveColors" {
        n181 = call "Curtin_SaveColor.vi"() -> ("New Color"=w208:string, "Good?"=w207:bool)  [unwired: 10 in]
        n182 = case shown="True" w207 {
          tunnel: w209 -> [_ w214]
          tunnel: w208 -> [_ w212]
          tunnel: [_ w213] -> _
          frame False {
          }
          frame True {
            n183 = for {
              tunnel: w214 -> [w219] mode=indexing
              tunnel: [w218] -> w217 mode=indexing
              n184 = Unbundle By Name(w219) -> ("Color"=w218:u32)
            }
            n185 = call "SettingsFiles.vi"("settings file name"=w212) -> ("file path"=w211:path)  [unwired: 9 in, 1 out]
            n186 = Write to Binary File(file (use dialog)=w211, data=w217, 5:FALSE ("prepend array or string size? (T)"), 9:T7."big-endian, network order" ("byte order (0:big-endian, network order)")) -> (error out=w213:errorcluster)  [unwired: 2 in, 2 out]
          }
        }
      }
      frame "setColors" {
        n187 = control-ref of="Files"() -> (w222:refnum<vi>)
        n188 = call "DefineColorPalette.vi"("Files in"=w221, "FileList"=w222) -> ("Files out"=w220:T1[])  [unwired: 9 in]
        n189 = call "Curtin_Undo.vi"("New Files"=w221, "Array in"=w224) -> ("Array out"=w223:cluster{"files":T1[]}[])  [unwired: 9 in]
      }
      frame "Fun" {
        n190 = call "FunArea.vi"("Old Files"=w225) -> ()  [unwired: 11 in]
      }
      frame "PlayIt" {
        n191 = call "PlayFile.vi"("Old Files"=w227) -> ()  [unwired: 11 in]
      }
      frame "Share" {
        n192 = call "Curtin1_Share.vi"("Files"=w229) -> ()  [unwired: 11 in]
      }
      frame "AppendTest" {
        n193 = global read "Mic_Global.vi" "Settings"() -> (w232:T12)
        n194 = call "Curtin1_DAQFiles.vi"("Settings"=w232, "Files in"=w233) -> ("Files out"=w231:T1[])  [unwired: 9 in]
        n195 = call "Curtin_Undo.vi"("New Files"=w233, "Array in"=w235) -> ("Array out"=w234:cluster{"files":T1[]}[])  [unwired: 9 in]
        n196 = flat-sequence {
          tunnel: w231 -> [_]
          frame #0 {
            n197 = call "BuildFileListFile.vi"("Task"=enum16{"BuildFile", "ReadFile"}."BuildFile") -> ()  [unwired: 9 in, 2 out]
          }
        }
      }
      frame "woodhouse" {
        n198 = call "Woodhouse.vi"("Files in"=w238) -> ("Files out"=w237:T1[])  [unwired: 10 in]
      }
      frame "SamZ" {
        n199 = call "SamZ_Format.vi"("Files in"=w241) -> ("Files out"=w240:T1[])  [unwired: 10 in]
      }
      frame "Folder" {
        n200 = for {
          tunnel: w244 -> [w250] mode=indexing
          tunnel: [w249] -> w243 mode=indexing if=w248
          n201 = Unbundle By Name(w250) -> ("Path"=w249:path, "Show?"=w248:bool)
        }
        n202 = for {
          tunnel: w243 -> [w247] mode=indexing
          n203 = Strip Path(path=w247) -> (stripped path=w246:path)  [unwired: 1 out]
          n204 = call "OpenFolder.vi"("LabVIEW Data Path"=w246) -> ()  [unwired: 11 in]
        }
      }
      frame "AppendAve" {
        n205 = local read "Complex Out"() -> (w255:cluster{dbl, "df":dbl, cdb[]}[])
        n206 = property on="View Type" class="Ring (strict)"() -> ("Value"=w253:u16)  [unwired: 2 in, 2 out]
        n207 = local read "# selected"() -> (w254:i32)
        n208 = call "SaveGroupAverages.vi"("nAverages"=w254, "Value"=w253, "Complex"=w255) -> ("New Path"=w251:path)  [unwired: 8 in]
        n209 = Not A Number/Path/Refnum?(number/path/refnum=w251) -> (NaN/Path/Refnum?=w252:bool)
        n210 = call "Curtin_Undo.vi"("New Files"=w257, "Array in"=w259) -> ("Array out"=w258:cluster{"files":T1[]}[])  [unwired: 9 in]
        n211 = case shown="False" w252 {
          tunnel: w257 -> [w264 w266]
          tunnel: [w263 w266] -> w256
          tunnel: w251 -> [w262 _]
          frame False {
            n212 = Build Array(w262) -> (w261:path[])
            n213 = call "Curtin1_AddTest.vi"("Old Files"=w264, "Selected Paths"=w261) -> ("New Files"=w263:T1[])  [unwired: 9 in]
            n214 = property on="View Type" class="Ring (strict)"("Val(Sgnl)"=0) -> ()  [unwired: 2 in, 2 out]
            n215 = call "BuildFileListFile.vi"("Task"=enum16{"BuildFile", "ReadFile"}."BuildFile") -> ()  [unwired: 9 in, 2 out]
          }
          frame True {
          }
        }
      }
      frame "Deselect" {
        n216 = for {
          tunnel: w269 -> [w272] mode=indexing
          tunnel: [w271] -> w268 mode=indexing
          n217 = Bundle By Name(cluster=w272, "Show?"=FALSE) -> (w271:T1)
        }
      }
      frame "SelectAll" {
        n218 = for {
          tunnel: w275 -> [w278] mode=indexing
          tunnel: [w277] -> w274 mode=indexing
          n219 = Bundle By Name(cluster=w278, "Show?"=TRUE) -> (w277:T1)
        }
      }
      frame "Clear" {
        n220 = call "Curtin_Undo.vi"("New Files"=w280, "Array in"=w281) -> ("Array out"=w279:cluster{"files":T1[]}[])  [unwired: 9 in]
        n221 = for {
          tunnel: w280 -> [w284] mode=indexing
          tunnel: [w284] -> w282 mode=indexing if=w283
          n222 = Unbundle By Name(w284) -> ("Show?"=w283:bool)
        }
      }
      frame "Clear All" {
        n223 = call "Curtin_Undo.vi"("New Files"=w285, "Array in"=w288) -> ("Array out"=w286:cluster{"files":T1[]}[])  [unwired: 9 in]
      }
      frame "Undo" {
        n224 = Array Size(array=w291) -> (size(s)=w289:i32)
        n225 = case shown="Default" w289 {
          tunnel: [w295 w299] -> w293
          tunnel: [w294 w296] -> w292
          tunnel: w291 -> [w295 w297]
          tunnel: w290 -> [w294 _]
          frame 0 {
          }
          frame Default {
            n226 = Delete From Array(array=w297) -> (deleted portion=w298:cluster{"files":T1[]}, array with subset deleted=w299:cluster{"files":T1[]}[])  [unwired: 2 in]
            n227 = Unbundle(w298) -> ("files"=w296:T1[])
          }
        }
      }
      frame "Left", "Right" {
        n228 = call "FadeLeftRight.vi"("Key"=w300) -> ()  [unwired: 11 in]
      }
      frame "BandEdit" {
        n229 = property on="Bands" class="Ring (strict)"() -> ("Strings []"=w310:string[], "Value"=w311:u16)  [unwired: 2 in, 2 out]
        n230 = for {
          tunnel: w308 -> [w317] mode=indexing
          tunnel: [w316] -> w307 mode=indexing if=w315
          n231 = Unbundle By Name(w317) -> ("Name"=w316:string, "Show?"=w315:bool)
        }
        n232 = Index Array(array=w310, index=w311) -> (element=w309:string)
        n233 = local read "FRF"() -> (w305:cluster{"x0":dbl, "df":dbl, dbl[]}[])
        n234 = Array Size(array=w307) -> (size(s)=w306:i32)
        n235 = call "ExtractBands.vi"("Task"=T8."Grab Lines", "lines"=w306, "plot in"=w305) -> ("plot out"=w304:cluster{dbl, "dt":dbl, "Y":dbl[]}[])  [unwired: 7 in, 1 out]
        n236 = call "BuildBandsList.vi"("Selected Band"=w309, "Average FRF"=w304) -> ("Name"=w314:string, "updated?"=w313:bool)  [unwired: 8 in]
        n237 = case shown="True" w313 {
          tunnel: w314 -> [_ w319]
          frame False {
          }
          frame True {
            n238 = call "Read-Save Bands.vi"("Task"=enum16{"Save", "Read", "List"}."List") -> ("Long names"=w320:string[])  [unwired: 7 in, 3 out]
            n239 = Search 1D Array(1D array=w320, element=w319) -> (index of element=w318:i32)  [unwired: 1 in]
            n240 = property on="Bands" class="Ring (strict)"("Strings []"=w320, "Value"=w318) -> ()  [unwired: 2 in, 2 out]
          }
        }
      }
      frame "resize" {
        n241 = property on="Show Notes" class="Bool"() -> ("Height"=w328:u32)  [unwired: 2 in, 2 out]
        n242 = property on="Pane 3" class="Pane"() -> ("Height"=w329:u32)  [unwired: 2 in, 2 out]
        n243 = control-ref of="FRF"() -> (w324:refnum<vi>)
        n244 = Add(x=u32 5, y=w328) -> (x+y=w327:u32)
        n245 = Divide(x=w329, y=w327) -> (x/y=w330:dbl)
        n246 = Round Toward -Infinity(1:w330) -> (0:w326:dbl)
        n247 = call "SetAxisLabels.vi"("WaveformGraph in"=w324) -> ("Bounds"=w322:T10, "Position"=w323:T11)  [unwired: 8 in, 1 out]
        n248 = property on="Files" class="Arr"("Number of Rows"=w326) -> ()  [unwired: 2 in, 2 out]
        n249 = property on="White Plots" class="Pict"("Position"=w323, "Draw Area Size"=w322) -> ()  [unwired: 2 in, 2 out]
      }
    }
    n250 = stacked-sequence {
      seq-local: ["Views" _ _ _] -> [_ w31 _ _]
      tunnel: w16 -> [w30 _ _ _]
      frame #0 {
        # "Update plot"
        n251 = local write "Files"(w30) -> ()
        n252 = control-ref of="FRF"() -> (w22:refnum<vi>)
        n253 = control-ref of="White Plots"() -> (w24:refnum<vi>)
        n254 = control-ref of="This VI"() -> (w28:refnum<vi>)
        n255 = call "Curtin1_Plot.vi"("Canvas 2"=w24, "Force YRescale"="Force YRescale", "Settings"="Views", "VI Refnum"=w28, "Files"=w30, "FRF"=w22) -> ("Complex Out"=→"Complex Out":cluster{dbl, "df":dbl, cdb[]}[], "size(s)"=→"# selected":i32, "Average FRF"=→"FRF":cluster{"x0":dbl, "df":dbl, dbl[]}[], "MJ Plot"=→"MJPlot":dbl[][])  [unwired: 2 in]
      }
      frame #1 {
        w35 = T2 6 items=["FRF", "rad phase unwrapped", "deg phase unwrapped", "rad phase wrapped", "deg phase wrapped", "White Plots", "MJ Map"] ("x")
        # "MJ Plot Stuff"
        n256 = property on="FRF" class="WFGraph (strict)"() -> ("YScale.Maximum"=w33:dbl, "YScale.Minimum"=w32:dbl)  [unwired: 2 in, 2 out]
        n257 = Unbundle By Name(w31) -> ("Plot"=w34:T2)
        n258 = Equal?(x=w35, y=w34) -> (x = y?=w36:bool)
        n259 = property on="Color Table" class="Enum (strict)"("Visible"=w36) -> ()  [unwired: 2 in, 2 out]
        n260 = property on="MJPlot" class="IntGraph (strict)"("Visible"=w36, "ZScale.Maximum"=w33, "ZScale.Minimum"=w32) -> ()  [unwired: 2 in, 2 out]
      }
      frame #2 {
        w37 = 0
        # "Populate lists (new templates?)"
        n261 = call "BuildTemplatePadLists.vi"() -> ("Templates"=w43:string[], "ScratchPads"=w38:string[])  [unwired: 8 in, 2 out]
        n262 = call "AllThingsColors.vi"() -> ("Possible Colors"=w41:string[])  [unwired: 11 in]
        n263 = local write "Force YRescale"(FALSE ("Force YRescale")) -> ()
        n264 = property on="ScratchPads" class="Ring (strict)"("Value"=w37, "Strings []"=w38) -> ()  [unwired: 2 in, 2 out]
        n265 = Build Array (concatenate)("Name Current...", w41) -> (w39:string[])
        n266 = property on="New Test" class="Ring (strict)"("Value"=w37, "Strings []"=w43) -> ()  [unwired: 2 in, 2 out]
        n267 = property on="Colors" class="Ring (strict)"("Strings []"=w39) -> ()  [unwired: 2 in, 2 out]
      }
      frame #3 {
        n268 = property on="Bands" class="Ring (strict)"() -> ("Value"=w45:u16)  [unwired: 2 in, 2 out]
        n269 = Greater Than 0?(x=w45) -> (x > 0?=w44:bool)
        n270 = property on="Excel" class="Bool"("Visible"=w44) -> ()  [unwired: 2 in, 2 out]
      }
    }
  }
  n271 = while {
    tunnel: w5 -> [w335]
    tunnel: w2 -> [w333]
    stop <- w334 stop-if-true
    n272 = event shown="[44] \"FRF\": Shortcut Menu Selection (User)" {
      selector: _ -> [_ _ _ _ _ _ _ _ _ _ _ _ _ _ _ _ _ _ _ _ _ _ _ _ _ _ _ _ _ _ _ _ _ _ _ _ _ _ _ _ _ _ _ _ _]
      dyn-events: _ -> [_ _ _ _ _ _ _ _ _ _ _ _ _ _ _ _ _ _ _ _ _ _ _ _ _ _ _ _ _ _ _ _ _ _ _ _ _ _ _ _ _ _ _ _ _]
      timeout: _ -> [_ _ _ _ _ _ _ _ _ _ _ _ _ _ _ _ _ _ _ _ _ _ _ _ _ _ _ _ _ _ _ _ _ _ _ _ _ _ _ _ _ _ _ _ _]
      tunnel: w335 -> [_ w336 w343 _ w354 w356 w359 w362 w366 w369 w372 w374 w378 w381 w384 w387 w390 w401 w416 _ w431 _ w449 _ w469 _ _ _ _ w501 _ _ w514 w538 _ w551 w556 w558 _ _ _ w568 w573 _ w580]
      tunnel: [_ w338 _ _ _ _ _ _ _ _ _ _ _ _ _ _ _ _ _ _ _ _ _ _ _ _ _ _ _ _ _ _ _ _ _ _ _ _ _ _ _ _ _ _ _] -> w334
      tunnel: w333 -> [_ w337 _ _ w353 w357 w358 w361 w364 w367 w370 w375 w377 w380 w382 w386 w388 w399 _ _ _ _ _ _ w468 _ _ _ _ _ _ _ w523 w537 _ w550 _ _ _ _ _ _ w574 _ _]
      tunnel: [_ _ _ _ _ _ _ _ _ _ _ _ _ _ _ _ _ _ _ _ _ _ _ _ _ _ _ _ _ _ _ _ _ _ _ _ _ _ _ _ _ _ _ w577 _] -> _
      tunnel: [_ _ _ _ _ _ _ _ _ _ _ _ _ _ _ _ _ _ _ w421 _ _ _ _ _ _ _ _ _ _ _ _ _ _ _ _ _ _ _ _ _ _ _ _ _] -> _
      event Timeout {
        n273 = event-data() -> ()  [unwired: 1 in, 3 out]
      }
      event Panel Close? {
        w338 = TRUE ("Discard?")
        n274 = event-data() -> ()  [unwired: 1 in, 4 out]
        n275 = call "Curtin_MouseBusy.vi"("VI in"=w337, "element"="Done", "queue in"=w336) -> ()  [unwired: 8 in, 1 out]
        n276 = event-data("Discard?"=w338) -> ()  [unwired: 1 in, 1 out]
      }
      event Key Down {
        n277 = event-data() -> ("VKey"=w344:T13, "PlatMods.Opt"=w342:bool, "PlatMods.Alt"=w341:bool)  [unwired: 1 in]
        n278 = Or(x=w342, y=w341) -> (x .or. y?=→"Ctrl":bool)
        n279 = case shown="\"Left\"" w344 {
          tunnel: w343 -> [_ w345 w347]
          frame Default {
          }
          frame "Left" {
            n280 = Enqueue Element(queue=w345, element="Left") -> ()  [unwired: 2 in, 3 out]
          }
          frame "Right" {
            n281 = Enqueue Element(queue=w347, element="Right") -> ()  [unwired: 2 in, 3 out]
          }
        }
      }
      event Key Up {
        n282 = event-data() -> ("PlatMods.Alt"=w351:bool, "PlatMods.Opt"=w350:bool)  [unwired: 1 in]
        n283 = Or(x=w351, y=w350) -> (x .or. y?=w349:bool)
        n284 = local write "Ctrl"(w349) -> ()
      }
      event Panel Resize {
        n285 = event-data() -> ()  [unwired: 1 in, 1 out]
        n286 = call "Curtin_MouseBusy.vi"("VI in"=w353, "element"="resize", "queue in"=w354) -> ()  [unwired: 8 in, 1 out]
      }
      event "Browse": Value Change {
        n287 = event-data() -> ()  [unwired: 1 in, 1 out]
        n288 = call "Curtin_MouseBusy.vi"("VI in"=w357, "element"="Browse", "queue in"=w356) -> ()  [unwired: 8 in, 1 out]
      }
      event "Search": Value Change {
        n289 = event-data() -> ()  [unwired: 1 in, 1 out]
        n290 = call "Curtin_MouseBusy.vi"("VI in"=w358, "element"="Search", "queue in"=w359) -> ()  [unwired: 8 in, 1 out]
      }
      event "deselect": Value Change {
        n291 = event-data() -> ()  [unwired: 1 in, 1 out]
        n292 = call "Curtin_MouseBusy.vi"("VI in"=w361, "element"="Deselect", "queue in"=w362) -> ()  [unwired: 8 in, 1 out]
      }
      event "select all": Value Change {
        n293 = event-data() -> ()  [unwired: 1 in, 1 out]
        n294 = call "Curtin_MouseBusy.vi"("VI in"=w364, "element"="SelectAll", "queue in"=w366) -> ()  [unwired: 8 in, 1 out]
      }
      event "Undo": Value Change {
        n295 = event-data() -> ()  [unwired: 1 in, 1 out]
        n296 = call "Curtin_MouseBusy.vi"("VI in"=w367, "element"="Undo", "queue in"=w369) -> ()  [unwired: 8 in, 1 out]
      }
      event "Redo": Value Change {
        n297 = event-data() -> ()  [unwired: 1 in, 1 out]
        n298 = call "Curtin_MouseBusy.vi"("VI in"=w370, "element"="Redo", "queue in"=w372) -> ()  [unwired: 8 in, 1 out]
      }
      event "Clear": Value Change {
        n299 = event-data() -> ()  [unwired: 1 in, 1 out]
        n300 = call "Curtin_MouseBusy.vi"("VI in"=w375, "element"="Clear", "queue in"=w374) -> ()  [unwired: 8 in, 1 out]
      }
      event "Files": Value Change {
        n301 = event-data() -> ()  [unwired: 1 in, 1 out]
        n302 = call "Curtin_MouseBusy.vi"("VI in"=w377, "element"="Update", "queue in"=w378) -> ()  [unwired: 8 in, 1 out]
      }
      event "Clear All": Value Change {
        n303 = event-data() -> ()  [unwired: 1 in, 3 out]
        n304 = call "Curtin_MouseBusy.vi"("VI in"=w380, "element"="Clear All", "queue in"=w381) -> ()  [unwired: 8 in, 1 out]
      }
      event "Lists": Value Change {
        n305 = event-data() -> ()  [unwired: 1 in, 1 out]
        n306 = call "Curtin_MouseBusy.vi"("VI in"=w382, "element"="Lists", "queue in"=w384) -> ()  [unwired: 8 in, 1 out]
      }
      event "Share": Value Change {
        n307 = event-data() -> ()  [unwired: 1 in, 1 out]
        n308 = call "Curtin_MouseBusy.vi"("VI in"=w386, "element"="Share", "queue in"=w387) -> ()  [unwired: 8 in, 1 out]
      }
      event "Colors": Value Change {
        n309 = event-data() -> ()  [unwired: 1 in, 2 out]
        n310 = case shown="Default" "Colors" {
          tunnel: w390 -> [w393 w398]
          tunnel: w388 -> [w391 w394]
          frame 0 {
            n311 = call "Curtin_MouseBusy.vi"("VI in"=w391, "element"="saveColors", "queue in"=w393) -> ()  [unwired: 8 in, 1 out]
          }
          frame Default {
            n312 = call "Curtin_MouseBusy.vi"("VI in"=w394, "element"="newColors", "queue in"=w398) -> ("queue out"=w396:refnum<queue>)  [unwired: 8 in]
            n313 = call "Curtin_MouseBusy.vi"("VI in"=w394, "element"="Update", "queue in"=w396) -> ()  [unwired: 8 in, 1 out]
          }
        }
      }
      event "Set Colors": Value Change {
        n314 = event-data() -> ()  [unwired: 1 in, 1 out]
        n315 = call "Curtin_MouseBusy.vi"("VI in"=w399, "element"="setColors", "queue in"=w401) -> ()  [unwired: 8 in, 1 out]
        n316 = disable-structure shown="Disabled" {
          disable-tunnel: _ -> [w402 _]
          frame Disabled {
            n317 = Enqueue Element(queue=w402, element="Update") -> ()  [unwired: 2 in, 3 out]
          }
          frame Enabled {
          }
        }
      }
      event "Views": Value Change {
        n318 = event-data() -> ("NewVal"=w404:T3)  [unwired: 1 in]
        n319 = Unbundle By Name(w404) -> ("X Scaling"=w411:bool, "Y Scaling"=w410:bool, "View Type"=w415:u16, "Edit"=w406:bool)
        n320 = global read "Mic_Global.vi" "View"() -> (w412:T9)
        n321 = Bundle By Name(cluster=w412, "Log X Axis"=w411, "dB scale"=w410) -> (w409:T9)
        n322 = Select(t="BandEdit" ("element"), s=w406, f="Update" ("element")) -> (s? t:f=w405:string)
        n323 = Enqueue Element(queue=w416, element=w405) -> ()  [unwired: 2 in, 3 out]
        n324 = global write "Mic_Global.vi" "View"(w409) -> ()
        n325 = Equal?(x=u16 1 ("View Type"), y=w415) -> (x = y?=w413:bool)
        n326 = property on="X_Low" class="DigNum (strict)"("Visible"=w413) -> ()  [unwired: 2 in, 2 out]
        n327 = property on="X_High" class="DigNum (strict)"("Visible"=w413) -> ()  [unwired: 2 in, 2 out]
      }
      event "Views.dB Range": Value Change {
        n328 = event-data() -> ()  [unwired: 1 in, 1 out]
        n329 = control-ref of="FRF"() -> (w420:refnum<vi>)
        n330 = property class="WFGraph (strict)"(reference=w420) -> (reference out=w423:refnum<vi>, error out=w422:errorcluster, "YScale.Maximum"=w426:dbl)  [unwired: 1 in]
        n331 = property on="dB Range" class="DigNum (strict)"() -> ("Value"=w425:dbl)  [unwired: 2 in, 2 out]
        n332 = Subtract(x=w426, y=w425) -> (x-y=w424:dbl)
        n333 = property class="WFGraph (strict)"(reference=w423, error in=w422, "YScale.Minimum"=w424) -> (reference out=w419:refnum<vi>, error out=w421:errorcluster)
        n334 = property on="Plot" class="Ring (strict)"() -> ("Value"=w418:T2)  [unwired: 2 in, 2 out]
        n335 = call "Curtin1_ReadWriteFRFGraphData.vi"("Type"=w418, "FRF"=w419, "Task"=enum16{"Read", "Save"}."Save") -> ()  [unwired: 6 in, 3 out]
      }
      event "Views.View Type": Value Change {
        n336 = event-data() -> ("NewVal"=w428:u16)  [unwired: 1 in]
        n337 = disable-structure shown="Disabled" {
          disable-tunnel: w431 -> [w432 _]
          frame Disabled {
            n338 = Enqueue Element(queue=w432, element="Update") -> ()  [unwired: 2 in, 3 out]
          }
          frame Enabled {
          }
        }
        n339 = Equal?(x=u16 1 ("View Type"), y=w428) -> (x = y?=w430:bool)
        n340 = property on="X_Low" class="DigNum (strict)"("Visible"=w430) -> ()  [unwired: 2 in, 2 out]
        n341 = property on="X_High" class="DigNum (strict)"("Visible"=w430) -> ()  [unwired: 2 in, 2 out]
        n342 = local write "Force YRescale"(TRUE ("Force YRescale")) -> ()
      }
      event Value Change {
        n343 = event-data() -> ("NewVal"=w434:T2, "OldVal"=w435:T2)  [unwired: 1 in]
        n344 = stacked-sequence {
          tunnel: w435 -> [w436 _]
          tunnel: w434 -> [_ w440]
          frame #0 {
            n345 = control-ref of="FRF"() -> (w438:refnum<vi>)
            n346 = call "Curtin1_ReadWriteFRFGraphData.vi"("Type"=w436, "FRF"=w438, "Task"=enum16{"Read", "Save"}."Save") -> ()  [unwired: 6 in, 3 out]
          }
          frame #1 {
            w441 = T2 5 items=["FRF", "rad phase unwrapped", "deg phase unwrapped", "rad phase wrapped", "deg phase wrapped", "White Plots"] ("y")
            # "There is a bug in LV so runs twice\none for changing Views and again\nfor changing scaling value..."
            n347 = control-ref of="FRF"() -> (w444:refnum<vi>)
            n348 = Equal?(x=w440, y=w441) -> (x = y?=w442:bool)
            n349 = call "Curtin1_ReadWriteFRFGraphData.vi"("Type"=w440, "FRF"=w444, "Task"=enum16{"Read", "Save"}."Read") -> ("y log?"=w447:bool, "x log?"=w446:bool, "dB"=w445:dbl)  [unwired: 6 in]
            n350 = property on="White Plots" class="Pict"("Visible"=w442) -> ()  [unwired: 2 in, 2 out]
            n351 = property on="dB Range" class="DigNum (strict)"("Value"=w445) -> ()  [unwired: 2 in, 2 out]
            n352 = property on="X Scaling" class="Bool (strict)"("Value"=w446) -> ()  [unwired: 2 in, 2 out]
            n353 = local write "Force YRescale"(TRUE ("Force YRescale")) -> ()
            n354 = property on="Y Scaling" class="Bool (strict)"("Val(Sgnl)"=w447) -> ()  [unwired: 2 in, 2 out]
          }
        }
      }
      event "White Plots": Mouse Move {
        n355 = event-data() -> ()  [unwired: 1 in, 1 out]
        n356 = property on="White Plots" class="Pict"() -> ("Width"=w450:u32, "Mouse"=w452:T14)  [unwired: 2 in, 2 out]
        n357 = Unbundle By Name(w452) -> ("Mouse Position.X"=w448:i32, "Mouse Modifiers.Button Down"=w451:bool)
        n358 = case shown="True" w451 {
          tunnel: w448 -> [_ w463]
          tunnel: w450 -> [_ w462]
          tunnel: w449 -> [_ w460]
          tunnel: w448 -> [_ w459]
          frame False {
          }
          frame True {
            n359 = local read "startX"() -> (w458:i32)
            n360 = Divide(x=w463, y=w462) -> ()  [unwired: 1 out]
            n361 = Subtract(x=w459, y=w458) -> (x-y=w457:i32)
            n362 = Enqueue Element(queue=w460, element="Update") -> ()  [unwired: 2 in, 3 out]
            n363 = Bundle(w457, "y"=0) -> (w454:cluster{i32, "y":i32})  [unwired: 1 in]
            n364 = Add(x=cluster{"x":dbl, "y":dbl}[] [{"x"=-400.0, "y"=200.0}, {"x"=400.0, "y"=200.0}] ("vanishing points"), y=w454) -> (x+y=w453:cluster{dbl, "y":dbl}[])
            n365 = global write "Perspective_Globals.vi" "vanishing points"(w453) -> ()
          }
        }
      }
      event "White Plots": Mouse Down; "White Plots": Mouse Enter {
        n366 = event-data() -> ()  [unwired: 1 in, 4 out]
        n367 = property on="White Plots" class="Pict" props=["Width", "Mouse"]() -> ("Mouse"=w466:T14)  [unwired: 2 in, 3 out]
        n368 = Unbundle By Name(w466) -> ("Mouse Position.X"=→"startX":i32, "Mouse Modifiers.Button Down"=w465:bool)
        n369 = global write "Perspective_Globals.vi" "Outlines?"(w465) -> ()
      }
      event "White Plots": Mouse Leave; "White Plots": Mouse Up {
        n370 = event-data() -> ()  [unwired: 1 in, 1 out]
        n371 = call "Curtin_MouseBusy.vi"("VI in"=w468, "element"="Update", "queue in"=w469) -> ()  [unwired: 8 in, 1 out]
        n372 = global write "Perspective_Globals.vi" "Outlines?"(FALSE ("Outlines?")) -> ()
      }
      event "Color Table": Value Change {
        n373 = event-data() -> ()  [unwired: 1 in, 6 out]
        n374 = call "ColorTables.vi"("Color Table"="Color Table") -> ("Color Table Out"=w474:u32[])  [unwired: 2 in]
        n375 = property on="MJPlot" class="IntGraph (strict)"("Color Table"=w474, "ZScale.Low Color"=u32 16777215 ("Z Scale.Low Color"), "ZScale.Interpolate Color"=TRUE ("Z Scale.Interpolate Color"), "ZScale.High Color"=u32 0 ("Z Scale.High Color")) -> ()  [unwired: 2 in, 2 out]
      }
      event "FRF": Mouse Move {
        n376 = event-data() -> ("CtlRef"=w481:refnum<vi>, "Coords"=w480:T5)  [unwired: 1 in]
        n377 = local read "Coords"() -> (w476:T5)
        n378 = property on="Plot" class="Ring (strict)"() -> ("Value"=w477:T2)  [unwired: 2 in, 2 out]
        n379 = case shown="True" "Mouse Down?" {
          tunnel: w481 -> [_ w488]
          tunnel: w480 -> [_ w484]
          tunnel: ["" ("Position") w487] -> w479
          tunnel: w477 -> [_ w485]
          tunnel: w476 -> [_ w483]
          frame False {
          }
          frame True {
            n380 = local read "Ctrl"() -> (w486:bool)
            n381 = call "Cursor Values.vi"("Plot"=w485, "option?"=w486, "Start Coord"=w483, "Coords"=w484, "WaveformGraph in"=w488) -> ("Position"=w487:string)  [unwired: 6 in]
          }
        }
        "Position" <- w479
      }
      event "FRF": Mouse Enter {
        n382 = event-data() -> ()  [unwired: 1 in, 1 out]
        n383 = local write "Mouse Down?"(TRUE ("Mouse Down?")) -> ()
      }
      event "FRF": Mouse Leave {
        n384 = event-data() -> ()  [unwired: 1 in, 1 out]
        n385 = local write "Mouse Down?"(FALSE ("Mouse Down?")) -> ()
        n386 = local write "Coords"(T5 {"Horizontal"=0, "Vertical"=0} ("Coords")) -> ()
        n387 = property on="FRF" class="WFGraph (strict)"("Active Cursor"=u32 0, "Cursor.Visible"=FALSE) -> ()  [unwired: 2 in, 2 out]
        n388 = property on="FRF" class="WFGraph (strict)"("Active Cursor"=u32 1, "Cursor.Visible"=FALSE) -> ()  [unwired: 2 in, 2 out]
      }
      event "FRF": Mouse Up {
        n389 = event-data() -> ("PlatMods.Shift"=w502:bool)  [unwired: 1 in]
        n390 = local write "Coords"(T5 {"Horizontal"=0, "Vertical"=0} ("Coords")) -> ()
        n391 = case shown="True" w502 {
          tunnel: w501 -> [_ w503]
          frame False {
          }
          frame True {
            n392 = Enqueue Element(queue=w503, element="Zoom") -> ()  [unwired: 2 in, 3 out]
          }
        }
        n393 = property on="FRF" class="WFGraph (strict)"("Active Cursor"=u32 0, "Cursor.Visible"=FALSE) -> ()  [unwired: 2 in, 2 out]
        n394 = property on="FRF" class="WFGraph (strict)"("Active Cursor"=u32 1, "Cursor.Visible"=FALSE) -> ()  [unwired: 2 in, 2 out]
      }
      event "FRF": Mouse Down {
        n395 = event-data() -> ("PlatMods.Ctrl"=w507:bool, "Coords"=→"Coords":T5)  [unwired: 1 in]
        n396 = Not(x=w507) -> (.not. x?=w505:bool)
        n397 = disable-structure shown="Disabled" {
          disable-tunnel: w505 -> [w508 _]
          frame Disabled {
            n398 = property on="FRF" class="WFGraph (strict)"("Active Cursor"=u32 0, "Cursor.Visible"=w508) -> ()  [unwired: 2 in, 2 out]
            n399 = property on="FRF" class="WFGraph (strict)"("Active Cursor"=u32 1, "Cursor.Visible"=w508) -> ()  [unwired: 2 in, 2 out]
          }
          frame Enabled {
          }
        }
      }
      event "FRF": Scale Range Change {
        n400 = event-data() -> ("CtlRef"=w512:refnum<vi>)  [unwired: 1 in]
        n401 = property on="Plot" class="Ring (strict)"() -> ("Value"=w511:T2)  [unwired: 2 in, 2 out]
        n402 = call "Curtin1_ReadWriteFRFGraphData.vi"("Type"=w511, "FRF"=w512, "Task"=enum16{"Read", "Save"}."Save") -> ()  [unwired: 6 in, 3 out]
      }
      event "New Test", "ScratchPads": Value Change {
        n403 = event-data() -> ()  [unwired: 1 in, 1 out]
        n404 = property on="ScratchPads" class="Ring (strict)"() -> ("Strings []"=w522:string[])  [unwired: 2 in, 2 out]
        n405 = property on="New Test" class="Ring (strict)"() -> ("Strings []"=w521:string[])  [unwired: 2 in, 2 out]
        n406 = Index Array(array=w522, index="ScratchPads") -> (element=w518:string)
        n407 = Index Array(array=w521, index="New Test") -> (element=w519:string)
        n408 = case shown="Default" "ScratchPads" {
          tunnel: w514 -> [_ w527]
          frame 0 {
            # "New Test"
          }
          frame Default {
            # "Clear old"
            n409 = Enqueue Element(queue=w527, element="Clear All") -> ()  [unwired: 2 in, 3 out]
          }
        }
        n410 = Not Equal To 0?(x="New Test") -> (x != 0?=w520:bool)
        n411 = Select(t=w519, s=w520, f=w518) -> (s? t:f=w517:string)
        n412 = flat-sequence {
          tunnel: w517 -> [_]
          frame #0 {
            w528 = 0
            n413 = local write "ScratchPads"(w528) -> ()
            n414 = local write "New Test"(w528) -> ()
          }
        }
        n415 = call "ScratchOrNew.vi"("Template"=w517) -> ("Success"=w525:bool, "Settings Out"=w524:T12)  [unwired: 9 in]
        n416 = case shown="True" w525 {
          tunnel: w524 -> [_ w532]
          tunnel: w514 -> [_ w531]
          tunnel: w523 -> [_ w530]
          frame False {
          }
          frame True {
            n417 = call "Curtin1_Acquire.vi"("MainVI"=w530, "Settings"=w532) -> ("Data?"=w529:bool)  [unwired: 7 in, 2 out]
            n418 = case shown="True" w529 {
              tunnel: w531 -> [_ w534]
              frame False {
                # "No data taken"
                n419 = call "Ask_delete.vi"() -> ()  [unwired: 12 in]
              }
              frame True {
                # "success"
                n420 = Enqueue Element(queue=w534, element="AppendTest") -> ()  [unwired: 2 in, 3 out]
              }
            }
          }
        }
      }
      event "Start": Value Change {
        n421 = event-data() -> ()  [unwired: 1 in, 1 out]
        n422 = call "Startup Wizard.vi"() -> ("analysis?"=w535:string, "Settings"=w536:T12)  [unwired: 10 in]
        n423 = case shown="\"acq\"" w535 {
          tunnel: w538 -> [w542 w546 _]
          tunnel: w537 -> [w541 _ _]
          tunnel: w536 -> [w540 _ _]
          frame "acq" {
            n424 = call "Curtin1_Acquire.vi"("MainVI"=w541, "Settings"=w540) -> ("Data?"=w539:bool)  [unwired: 7 in, 2 out]
            n425 = case shown="True" w539 {
              tunnel: w542 -> [_ w544]
              frame False {
                # "No data taken"
                n426 = call "Ask_delete.vi"() -> ()  [unwired: 12 in]
              }
              frame True {
                n427 = Enqueue Element(queue=w544, element="AppendTest") -> ()  [unwired: 2 in, 3 out]
              }
            }
          }
          frame "analysis" {
            n428 = Enqueue Element(queue=w546, element="Preload") -> ()  [unwired: 2 in, 3 out]
          }
          frame Default {
          }
        }
      }
      event "Help": Value Change {
        n429 = event-data() -> ()  [unwired: 1 in, 1 out]
        n430 = fn#1354() -> (1:w548:bool)  [unwired: 1 out]
        n431 = Not(x=w548) -> (.not. x?=w547:bool)
        n432 = Control Help Window(1:w547) -> ()  [unwired: 1 in]
      }
      event "Preferences": Value Change {
        n433 = event-data() -> ()  [unwired: 1 in, 1 out]
        n434 = call "Curtin_MouseBusy.vi"("VI in"=w550, "element"="Preferences", "queue in"=w551) -> ()  [unwired: 8 in, 1 out]
      }
      event "Settings": Value Change {
        w552 = u16 0 items=["Settings...", "Preferences", "Templates", "Calibrations"] ("Settings")
        n435 = event-data() -> ()  [unwired: 1 in, 1 out]
        n436 = Index Array(array=string[] ["", "Preferences", "Templates", "Calibrations", "LiveView", "MotorControl"], index="Settings") -> (element=w553:string)
        n437 = Enqueue Element(queue=w556, element=w553) -> ()  [unwired: 2 in, 3 out]
        n438 = local write "Settings"(w552) -> ()
      }
      event "zoom": Value Change {
        n439 = event-data() -> ()  [unwired: 1 in, 1 out]
        n440 = Enqueue Element(queue=w558, element="Zoom") -> ()  [unwired: 2 in, 3 out]
      }
      event "email": Value Change {
        n441 = event-data() -> ()  [unwired: 1 in, 1 out]
        n442 = call-poly <vilib>:"Open URL in Default Browser.vi"("URL"="https://sites.google.com/view/oberlinacoustics/contactbug-reports") -> ()  [unwired: 5 in, 2 out]
      }
      event "About": Value Change {
        n443 = event-data() -> ()  [unwired: 1 in, 1 out]
        n444 = call "ObieHelp.vi"() -> ()  [unwired: 12 in]
      }
      event "Interpret": Value Change {
        n445 = event-data() -> ()  [unwired: 1 in, 1 out]
        n446 = property on="Bands" class="Ring (strict)"() -> ("Value"=w562:u16)  [unwired: 2 in, 2 out]
        n447 = local read "FRF"() -> (w560:cluster{"x0":dbl, "df":dbl, dbl[]}[])
        n448 = case shown="Default" w562 {
          tunnel: [w563 w564] -> w561
          tunnel: w560 -> [w563 w566]
          frame 0 {
          }
          frame Default {
            n449 = Array Size(array=w566) -> (size(s)=w567:i32)
            n450 = expression code="x*2/3"(w567) -> (w565:i32)
            n451 = Split 1D Array(array=w566, index=w565) -> (second subarray=w564:cluster{"x0":dbl, "df":dbl, dbl[]}[])  [unwired: 1 out]
          }
        }
        n452 = call "Explainations.vi"("FRF"=w561) -> ()  [unwired: 11 in]
      }
      event "Fun": Value Change {
        n453 = event-data() -> ()  [unwired: 1 in, 1 out]
        n454 = Enqueue Element(queue=w568, element="Fun") -> ()  [unwired: 2 in, 3 out]
      }
      event "microphone": Value Change {
        (unwired) "Preferences" ("element")
        n455 = event-data() -> ()  [unwired: 1 in, 1 out]
        n456 = call "Curtin_MouseBusy.vi"("VI in"=w574, "element"="LiveView", "queue in"=w573) -> ()  [unwired: 8 in, 1 out]
        n457 = property on="Device" class="Ring (strict)"("Strings []"=string[] ["Initializing..."] ("Strings [4]"), "Value"=0) -> ()  [unwired: 2 in, 2 out]
      }
      event "FRF": Shortcut Menu Activation? {
        n458 = event-data() -> ("MenuRef"=w578:refnum<k9>)  [unwired: 1 in]
        n459 = property on="Bands" class="Ring (strict)"() -> ("Value"=w575:u16)  [unwired: 2 in, 2 out]
        n460 = property on="View Type" class="Ring (strict)"() -> ("Value"=w576:u16)  [unwired: 2 in, 2 out]
        n461 = call "GenerateMenuItems.vi"("Bands"=w575, "View Type"=w576, "Menu in"=w578) -> ("error out"=w577:errorcluster)  [unwired: 8 in]
        n462 = event-data() -> ()  [unwired: 2 in, 1 out]
      }
      event "FRF": Shortcut Menu Selection (User) {
        n463 = event-data() -> ("CtlRef"=w579:refnum<vi>, "ItemTag"=w581:string)  [unwired: 1 in]
        n464 = case shown="\"savePlot\"" w581 {
          tunnel: w580 -> [_ w582 _ _ _ w592 w595 _ _ w598 w600 w602 _]
          tunnel: w579 -> [_ _ w588 w589 _ _ _ _ _ _ _ _ _]
          frame Default {
          }
          frame "toggleCentroids" {
            n465 = global read "Mic_Global.vi" "View"() -> (w586:T9)
            n466 = Unbundle By Name(w586) -> ("Centroids?"=w587:bool)
            n467 = Enqueue Element(queue=w582, element="Update") -> ()  [unwired: 2 in, 3 out]
            n468 = Not(x=w587) -> (.not. x?=w585:bool)
            n469 = Bundle By Name(cluster=w586, "Centroids?"=w585) -> (w584:T9)
            n470 = global write "Mic_Global.vi" "View"(w584) -> ()
          }
          frame "savePlot" {
            n471 = call "ExportPlots.vi"("WaveformGraph in"=w588) -> ()  [unwired: 11 in]
          }
          frame "copyImage" {
            n472 = call "GrabPlotImage.vi"("WaveformGraph in"=w589) -> ()  [unwired: 11 in]
          }
          frame "autoScale" {
            n473 = property on="dB Range" class="DigNum (strict)"() -> ("Value"=w591:dbl)  [unwired: 2 in, 2 out]
            n474 = call "AutoscaleYaxis.vi"("Has Coherence in plot?"=FALSE, "dB Range"=w591) -> ()  [unwired: 10 in]
          }
          frame "Folder" {
            n475 = Enqueue Element(queue=w592, element="Folder") -> ()  [unwired: 2 in, 3 out]
          }
          frame "saveGroup" {
            n476 = Enqueue Element(queue=w595, element="AppendAve") -> ()  [unwired: 2 in, 3 out]
          }
          frame "FontAdjust" {
            n477 = control-ref of="FRF"() -> (w596:refnum<vi>)
            n478 = call "Ask_Font.vi"("WaveformGraph in"=w596) -> ()  [unwired: 11 in]
          }
          frame "MATLAB" {
            n479 = control-ref of="FRF"() -> (w597:refnum<vi>)
            n480 = call "MATLAB.vi"("Graph"=w597) -> ()  [unwired: 10 in, 1 out]
          }
          frame "WOOD" {
            n481 = Enqueue Element(queue=w598, element="woodhouse") -> ()  [unwired: 2 in, 3 out]
          }
          frame "SAM" {
            n482 = Enqueue Element(queue=w600, element="SamZ") -> ()  [unwired: 2 in, 3 out]
          }
          frame "PLAY" {
            n483 = Enqueue Element(queue=w602, element="PlayIt") -> ()  [unwired: 2 in, 3 out]
          }
          frame "Trends" {
            n484 = control-ref of="FRF"() -> (w606:refnum<vi>)
            n485 = property on="Bands" class="Ring (strict)"() -> ("Value"=w605:u16)  [unwired: 2 in, 2 out]
            n486 = Not Equal To 0?(x=w605) -> (x != 0?=w604:bool)
            n487 = call "PlotBandsAgainstRun.vi"("Bands?"=w604, "Graph"=w606) -> ()  [unwired: 10 in]
          }
        }
      }
    }
  }
  n488 = disable-structure shown="Default" {
    disable-tunnel: [_ TRUE] -> w10
    frame condition #0 (active) {
    }
    frame condition #1 {
    }
  }
  n489 = property on="Position" class="Str"("Text.FontBold"=w10) -> ()  [unwired: 2 in, 2 out]
  n490 = disable-structure shown="RUN_TIME_ENGINE==True" {
    disable-tunnel: w9 -> [_ _]
    frame condition #0 (active) {
    }
    frame condition #1 {
      # "Stop everytng from running"
      n491 = control-ref of="This VI"() -> (w609:refnum<vi>)
      n492 = property class="VI"("FP.State"=T15."Closed" ("Front Panel Window:State")) -> (error out=w608:errorcluster)  [unwired: 2 in, 1 out]
      n493 = invoke class="VI" method="Abort VI"(reference=w609, error in=w608) -> ()  [unwired: 1 in, 3 out]
    }
  }
